vi "CreateArrayScripter.vi"(1 "Ctl Refnum":refnum<vi>, 2 "LVClassLibrary Ref":refnum<vi>) -> (0 "Scripter Out":refnum<class "ArrayElementScripter.lvclass">)   [LabVIEW 2021, in "MemberVICreation.lvlib" / "ArrayElementScripter.lvclass"]
uses:
  <resource>/Framework/Providers/LVClassLibrary/NewAccessors/ArrayElementScripter/ArrayElementScripter.lvclass
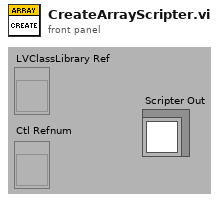
[diagram p1: front panel]
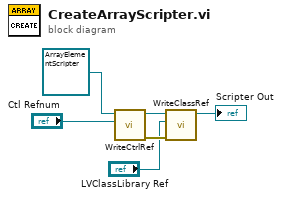
[diagram p0: block diagram]
diagram:
  n1 = call-dynamic "WriteCtrlRef.vi"("Ctl Refnum"="Ctl Refnum", "BaseAccessorScripter in"=refnum<class "ArrayElementScripter.lvclass"> refnum ("Scripter Out")) -> ("error out"=w6:errorcluster, "BaseAccessorScripter out"=w5:refnum<class "ArrayElementScripter.lvclass">)  [unwired: 1 in, 7 out]
  n2 = call-dynamic "WriteClassRef.vi"("error in (no error)"=w6, "LVClassLibrary Ref"="LVClassLibrary Ref", "BaseAccessorScripter in"=w5) -> ("BaseAccessorScripter out"=→"Scripter Out":refnum<class "ArrayElementScripter.lvclass">)  [unwired: 8 out]
